vi "PhotoeyeOut.vi"(8 "Hard Stop":bool, 9 "MotorPower":dbl, 10 "Button":bool, 11 "MotorIn":dbl) -> (0 "Complete":bool, 3 "MotorOut":dbl)   [LabVIEW 2015]
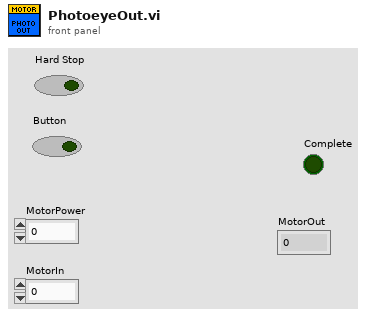
[diagram p1: front panel]
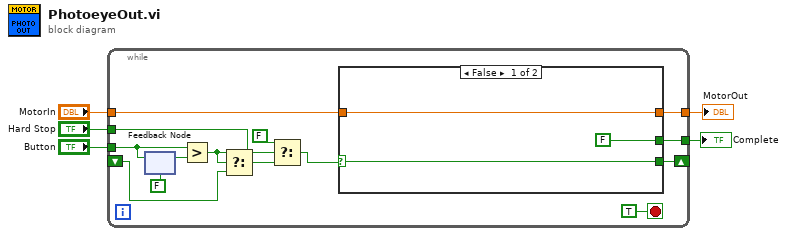
[diagram p0: block diagram]
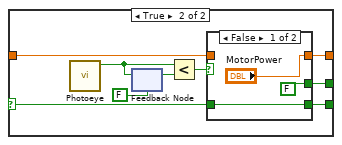
[diagram p2: hidden frame]
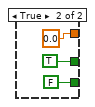
[diagram p3: hidden frame]
diagram:
  n1 = while {
    tunnel: "Button" -> [w11]
    tunnel: [w19] -> w4
    tunnel: "MotorIn" -> [w18]
    shift-right: [w13] -> _
    shift-left: _ -> [w12]
    tunnel: [w10] -> w2
    tunnel: "Hard Stop" -> [w8]
    stop <- TRUE stop-if-true
    n2 = feedback-in #1(w11) -> ()
    n3 = feedback #1(FALSE) -> (w16:bool)
    n4 = Greater?(x=w11, y=w16) -> (0:w14:bool)
    n5 = Select(t=w14, s=w14, f=w12) -> (s? t:f=w9:bool)
    n6 = Select(t=FALSE, s=w8, f=w9) -> (s? t:f=w6:bool)
    n7 = case shown="False" w6 {
      selector: w6 -> [w21 w30]
      tunnel: [w22 w31] -> w19
      tunnel: w18 -> [w22 w28]
      tunnel: [w21 w29] -> w13
      tunnel: [FALSE w27] -> w10
      frame False {
      }
      frame True {
        n8 = call "Photoeye.vi"() -> ("BeamBroken?"=w23:bool)  [unwired: 11 in]
        n9 = feedback #2(FALSE) -> (w25:bool)
        n10 = feedback-in #2(w23) -> ()
        n11 = Less?(x=w23, y=w25) -> (x < y?=w24:bool)
        n12 = case shown="False" w24 {
          tunnel: ["MotorPower" 0.0 ("MotorIn")] -> w31
          tunnel: w30 -> [w34 _]
          tunnel: [w34 FALSE] -> w29
          tunnel: w28 -> [_ _]
          tunnel: [FALSE TRUE] -> w27
          frame False {
          }
          frame True {
          }
        }
      }
    }
  }
  "MotorOut" <- w4
  "Complete" <- w2
